vi "Write Frame.vi"(7 "OpCode":T1, 8 "error in (no error)":errorcluster, 9 "Timeout ms":i32, 10 "Payload":string, 11 "WebsocketStream in":refnum<class "WebsocketStream.lvclass">) -> (0 "error out":errorcluster, 1 "Remaining  Timeout":i32, 3 "WebsocketStream out":refnum<class "WebsocketStream.lvclass">)   [LabVIEW 2020, in "Stream-Websocket.lvlib" / "WebsocketStream.lvclass"]
uses:
  WebsocketStream.lvclass
  OpCode.ctl
  WebsocketStream.lvclass/WebsocketStream.ctl
  Stream-Websocket.lvlib
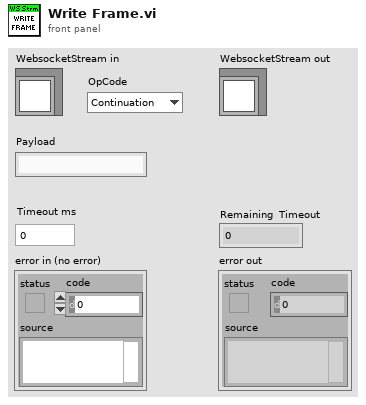
[diagram p1: front panel]
types:
  T1 = typedef "Stream-Websocket.lvlib/OpCode.ctl" = enum8{"Continuation", "Text", "Binary", "Reserved3", "Reserved4", "Reserved5", "Reserved6", "Reserved7", "Close", "Ping", "Pong", "ReservedB", "ReservedC", "ReservedD", "ReservedE", "ReservedF"}
  T2 = typedef "Stream-Websocket.lvlib/Message Frame.ctl" = cluster{"FIN":bool, "RSV1":bool, "RSV2":bool, "RSV3":bool, "MASK":bool, "OpCode":T1, "Length":u64, "MaskingKey":u8[], "Payload":string}
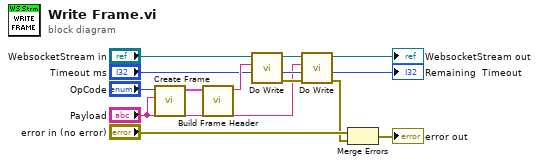
[diagram p0: block diagram]
diagram:
  n1 = call "Create Frame.vi"("Payload"="Payload", "OpCode"="OpCode") -> ("Message Frame"=w13:T2)  [unwired: 9 in]
  n2 = call "Build Frame Header.vi"("Message Frame"=w13) -> ("Header"=w11:string)  [unwired: 10 in]
  n3 = call "Do Write.vi"("Timeout ms"="Timeout ms", "Data"=w11, "WebsocketStream in"="WebsocketStream in") -> ("error out"=w9:errorcluster, "Remaining  Timeout"=w7:i32, "WebsocketStream out"=w8:refnum<class "WebsocketStream.lvclass">)  [unwired: 6 in]
  n4 = call "Do Write.vi"("error in (no error)"=w9, "Timeout ms"=w7, "Data"="Payload", "WebsocketStream in"=w8) -> ("error out"=w2:errorcluster, "Remaining  Timeout"=→"Remaining  Timeout":i32, "WebsocketStream out"=→"WebsocketStream out":refnum<class "WebsocketStream.lvclass">)  [unwired: 5 in]
  n5 = Merge Errors("error in (no error)", w2) -> (→"error out":errorcluster)
